vi "Dashboard Main.vi"() -> ()   [LabVIEW 2017]
uses:
  Shared/AutonomousRoutine.ctl
  Shared/RobotPosition.ctl
  Shared/AutoRoutineSelector.ctl
  <vilib>/Rock Robotics/WPI/DriverStation/WPI_DriverStationAllianceInfo.ctl
  <vilib>/Utility/miscctls.llb/LVRowAndColumnTypeDef.ctl
  <vilib>/event_ctls.llb/eventvkey.ctl
  <vilib>/Rock Robotics/Network Tables/NT Read Numeric Array.vi
  <vilib>/Rock Robotics/WPI/Dashboard/WPI_DashboardLogging Global.vi
  <vilib>/Rock Robotics/Network Tables/NT Write Boolean.vi
  <vilib>/Rock Robotics/Network Tables/NT Write Numeric Array.vi
panel:
  in  "Camera Settings Right":T1={"Frame Rate"=30, "Compression"=30, "Size"=1, "DB Camera Config"=FALSE} {"Frame Rate" scale=1.0..30.0; "Compression" scale=100.0..-1.0; "Size" items=["640x480", "320x240", "160x120"]}
  in  "Camera Name Right":string(combo)="No Camera Selection"
  out "Camera Info":cluster{"Mbps LED":bool, "Mbps":dbl, "fps":dbl} {"fps" format="%#.1g"; "Mbps" format="%#.1g"}
  in  "Camera Settings":T1={"Frame Rate"=30, "Compression"=30, "Size"=1, "DB Camera Config"=FALSE} {"Frame Rate" scale=1.0..30.0; "Compression" scale=100.0..-1.0; "Size" items=["640x480", "320x240", "160x120"]}
  in  "TCP":refnum<k5>
  in  "Rec Mode":enum32{"Stop", "Record", "Playback"}(radio)
  out "Robot IP":string
  out "Image Message":string="Timeout in Camera Communications"
  in  "Dashboard Tab":T2(tab)
  in  "Select Auto":string(combo)="Select Autonomous ..."
  out "NT Connection":bool
  out "MotorChart R":cluster{"Numeric":dbl, "Numeric":dbl}(graph)
  out "MotorChart L":cluster{"Numeric":dbl, "Numeric":dbl}(graph)
  out "MotorSliders R":cluster{"MotorSlide1":dbl, "MotorSlide2":dbl} {"MotorSlide2" scale=-1.0..1.0 scale format="%#_2e"; "MotorSlide1" scale=-1.0..1.0 scale format="%#_2e"}
  out "MotorSliders L":cluster{"MotorSlide1":dbl, "MotorSlide2":dbl} {"MotorSlide2" scale=-1.0..1.0 scale format="%#_2e"; "MotorSlide1" scale=-1.0..1.0 scale format="%#_2e"}
  out "Gyro":dbl(knob) scale=0.0..360.0
  out "JS1 Z":dbl(slide) scale=-1.0..1.0 scale format="%#_2e"
  out "JS1 Graph":cluster{"X":dbl, "Y":dbl}[](graph)
  out "JS1 Buttons":T3
  out "JS2 Z":dbl(slide) scale=-1.0..1.0 scale format="%#_2e"
  out "JS2 Graph":cluster{"X":dbl, "Y":dbl}[](graph)
  out "JS2 Buttons":T3
  out "Mode":T4(ring)=enum."Auto Disabled"
  in  "Battery Number":string
  out "Camera Image Right":T5(plugin-control)
  in  "DB/String 9":string
  in  "DB/String 8":string
  in  "DB/String 7":string
  in  "DB/String 6":string
  in  "DB/String 5":string
  in  "DB/String 4":string
  in  "DB/String 3":string
  in  "DB/String 2":string
  in  "DB/String 1":string
  in  "DB/String 0":string
  in  "DB/Slider 0":dbl(slide) scale=0.0..5.0
  in  "DB/Slider 1":dbl(slide) scale=0.0..5.0
  in  "DB/Slider 2":dbl(slide) scale=0.0..5.0
  in  "DB/Slider 3":dbl(slide) scale=0.0..5.0
  out "DB/LED 3":bool
  out "DB/LED 2":bool
  out "DB/LED 1":bool
  out "DB/LED 0":bool
  in  "DB/Button 3":bool
  in  "DB/Button 2":bool
  in  "DB/Button 1":bool
  in  "DB/Button 0":bool caption="New Name"
  in  "Routine":T6 items=["Definately Switch", "Definately Scale", "Switch if in front, else scale", "Scale if in front, else switch", "Switch if in front, else nothing", "Scale if in front, else nothing", "Drive across line"]
  in  "RR":T7
  in  "RL":T7
  in  "LR":T7
  in  "Position":T8
  in  "LL":T7
  out "Our Right Team Switch":bool
  out "Our Left Team Switch":bool
  out "Center Right Scale":bool
  out "Center Left Scale":bool
  out "Opponent Right Switch":bool
  out "Opponent Left Switch":bool
  in  "Test Slider":dbl(slide) scale=0.0..100.0 scale format="%#_3g"
  in  "On/Off":bool caption="Solenoid"
  in  "Test Name":u16(ring) items=["Select the test to run..."]
  in  "Test Tree":string(tree)
  in  "Motor":cluster{"Value":dbl, "Enable":bool} {"Value" scale=-1.0..1.0 scale format="%#_3g"}
  out "Progress":T9 {"Test Progress" scale=0.0..100.0}
  in  "Rev/Fwd":cluster{"Forward":bool, "Reverse":bool}
  in  "Test Ring":u16(ring) items=["Monochrome", "Color"]
  out "Cmd Status":string
  in  "Execute Command":bool
  in  "Command Params":string[][](table)
  in  "Command Selection":i32(listbox)
  in  "CheckList":i32(listbox)
  out "Tree":string(tree)
  out "Camera Image":T5(plugin-control)
  out "Background":bool
  in  "Camera Name":string(combo)="No Camera Selection"
  # "HW"
  # "HW"
  # "Joysticks"
  # "Drive Motors"
  # "Front"
  # "Right"
  # "Left"
  # "Back"
  # "Opponent Switch"
  # "Center Scale"
  # "Our Team Switch"
  # "1"
  # "2"
  # "3"
  # "4"
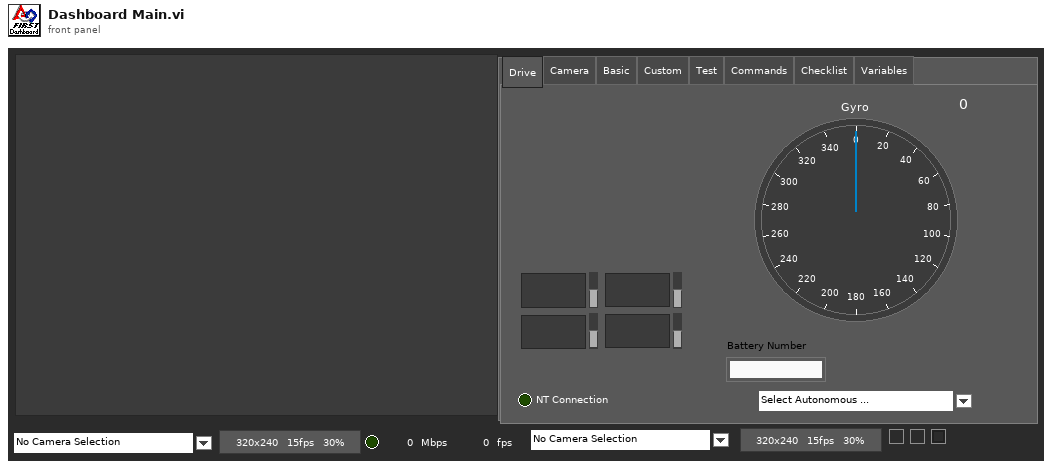
[diagram p1: front panel]
types:
  T1 = cluster{"Frame Rate":i32, "Compression":i32, "Size":u16, "DB Camera Config":bool}
  T2 = enum32{"Drive", "Camera", "Basic", "Custom", "Test", "Commands", "Checklist", "Variables"}
  T3 = cluster{bool, bool, bool, bool, bool, bool, bool, bool, bool, bool, bool, bool}
  T4 = enum8{"Tele-Op Disabled", "Tele-Op Enabled", "Auto Disabled", "Auto Enabled", "Test Disabled", "Test Enabled", "Disconnected", "No Code", "E-Stop"}
  T5 = typedef "IMAQ Image.ctl" = refnum<image>
  T6 = typedef "AutoRoutineSelector.ctl" = u16
  T7 = typedef "AutonomousRoutine.ctl" = enum16{"Score Scale", "Score Switch"}
  T8 = typedef "RobotPosition.ctl" = enum16{"1", "2", "3", "4"}
  T9 = cluster{"Test Progress":u8, "Test Progress Text":string}
  T10 = cluster{"Save Path":path, "Interval (s)":dbl, "Keep":i32}
  T11 = typedef "Image Type" = u32
  T12 = cluster{"IDs":cluster{"RPC field ID":u16, "Unique ID":u16}, "String":string}
  T13 = cluster{"Error Strings":string, "Disable Counts":cluster{u16, u16}, "Rail Faults":cluster{u16, u16, u16}, "Robot IP":string, "DB Mode":u8, "Event Info":cluster{"Name":string, "Type":u8, "Number":u16, "Replay":u8}}
  T14 = cluster{"Storage":cluster{"Disk Free":u64, "RAM Block":u32, "RAM free":u32}, "CPU Utilization":cluster{"CPU % ISR":sgl, "CPU % Time Crit":sgl, "CPU % Timed Str":sgl, "CPU % High":sgl, "CPU % Above":sgl, "CPU % Normal":sgl, "CPU % Low":sgl}, "CAN":cluster{"% Bus Utilization":sgl, "Bus Off Cnt":u32, "TX_FIFO Full Cnt":u32, "Receive Error Cnt":u8, "Transmit Error Cnt":u8}, "HID":cluster{"HID Outputs":u32, "Rumble Low":u16, "Rumble High":u16}[]}
  T15 = cluster{"Status bits":cluster{"Test Mode":bool, "Autonomous":bool, "Enabled":bool, "Code Start":bool, "Brownout":bool, "Reserved 2":bool, "Reserved 3":bool, "E-Stop":bool}, "Code Trace":cluster{"Disabled":bool, "TeleOp":bool, "Auto":bool, "Test":bool}, "Controller Type":enum16{"unknown", "cRIO", "roboRio"}, "Code?":enum16{"unknown", "noCode", "code"}, "Battery V":dbl}
  T16 = cluster{"Control Bits":cluster{"TestMode":bool, "Autonomous":bool, "Enabled":bool, "FMS Present":bool, bool, bool, bool, "E-Stop":bool}, "Team Station ":u8, "Countdown":sgl, "Joystick Values":cluster{"Axes":dbl[], "Buttons":bool[], "POVs":i16[]}[]}
  T17 = cluster{"Axes":dbl[], "Buttons":bool[], "POVs":i16[]}[]
  T18 = cluster{"Axes":dbl[], "Buttons":bool[], "POVs":i16[]}
  T19 = cluster{"Buttons[0]":bool, "Buttons[1]":bool, "Buttons[2]":bool, "Buttons[3]":bool, "Buttons[4]":bool, "Buttons[5]":bool, "Buttons[6]":bool, "Buttons[7]":bool, "Buttons[8]":bool, "Buttons[9]":bool, "Buttons[10]":bool, "Buttons[11]":bool}
  T20 = cluster{"Camera Image":refnum<vi>, "Dashboard Tab":refnum<vi>, "Background":refnum<vi>, "Rec Mode":refnum<vi>, "Test Slider":refnum<vi>, "On/Off ":refnum<vi>, "Test Ring":refnum<vi>, "Rev/Fwd":refnum<vi>, "Test Name":refnum<vi>, "Motor":refnum<vi>, "Progress":refnum<vi>, "CheckList":refnum<vi>, "Tree":refnum<vi>, "Test Tree":refnum<vi>, "Command Params":refnum<vi>, "Command Selection":refnum<vi>, "Execute Command":refnum<vi>, "Cmd Status":refnum<vi>, "Camera Settings":refnum<vi>, "Camera Name":refnum<vi>, "Camera Info":refnum<vi>, "Camera Settings Right":refnum<vi>, "Camera Name Right":refnum<vi>, "Camera Image Right":refnum<vi>}
  T21 = cluster{"Camera Name":string, string, "Saved DB Images Info":cluster{"Save Path":path, "Interval (s)":dbl, "Keep":i32}}
  T22 = cluster{"Camera Name Right":string, string, "Saved DB Images Info":cluster{"Save Path":path, "Interval (s)":dbl, "Keep":i32}}
  T23 = typedef "WPI_DriverStationAllianceInfo.ctl" = enum16{"Red", "Blue", "Invalid"}
  T24 = cluster{"Operation":enum16{"Update", "Clear"}, "Color Box":u32}[]
  T25 = typedef "eventvkey.ctl" = enum16{"ASCII", "Enter", "Return", "Shift", "Ctrl", "Alt", "Cmd", "Opt", "Caps", "NumLock", "Clear", "Break", "Up", "Down", "Left", "Right", "Insert", "Delete", "Home", "End", "PageUp", "PageDown", "Escape", "Help", "Pause", "ScrollLock", "F1", "F2", "F3", "F4", "F5", "F6", "F7", "F8", "F9", "F10", "F11", "F12", "F13", "F14", "F15", "F16", "F17", "F18", "F19", "F20", "F21", "F22", "F23", "F24", "Play", "VolumeUp", "VolumeDown", "Mute", "Two Byte Char"}
  T26 = cluster{"Image Size":bool, "Image Type":bool, "Pixel Value":bool, "ROI Information":bool, "Zoom Factor":bool}
  T27 = cluster{"Operation":enum16{"Update", "Clear"}, "Color Box":u32}
  T28 = typedef "LVRowAndColumnTypeDef.ctl" = cluster{"Row":i32, "Column":i32}
  T29 = cluster{"Shift":bool, "Ctrl":bool, "Alt":bool, "Cmd":bool, "Opt":bool}
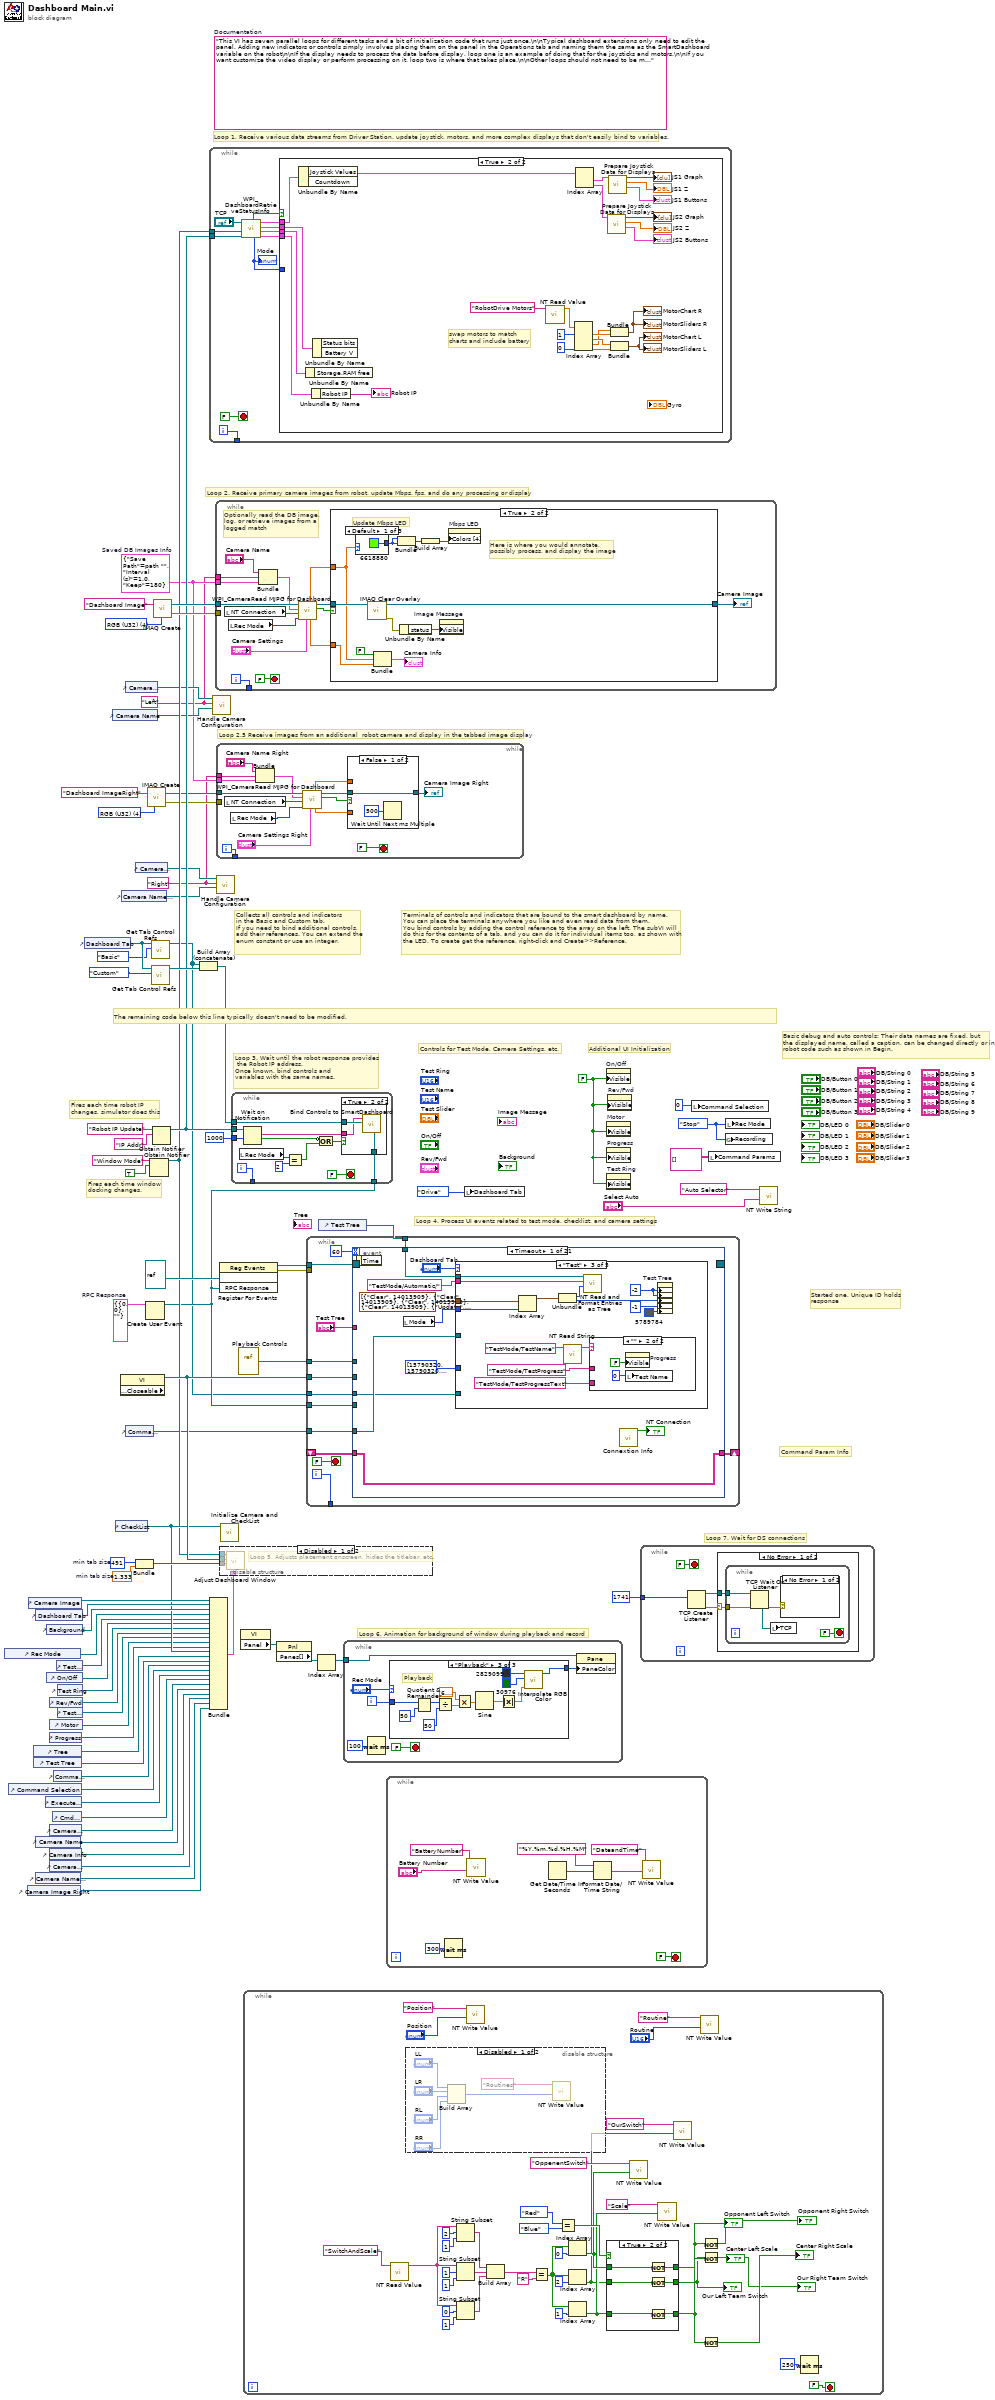
[diagram p0: block diagram]
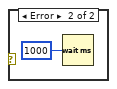
[diagram p6: hidden frame]
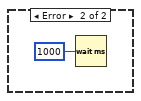
[diagram p7: hidden frame]
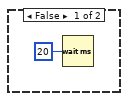
[diagram p8: hidden frame]
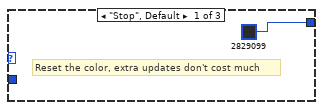
[diagram p9: hidden frame]
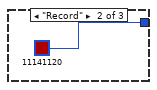
[diagram p10: hidden frame]
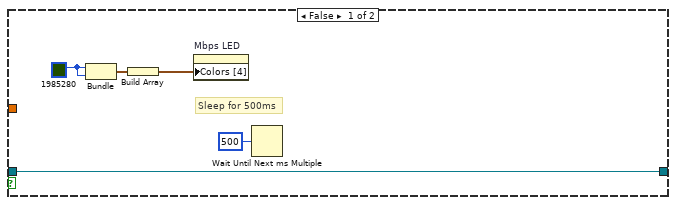
[diagram p12: hidden frame]
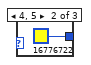
[diagram p13: hidden frame]
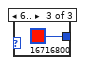
[diagram p14: hidden frame]
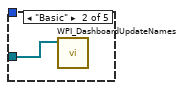
[diagram p16: hidden frame]
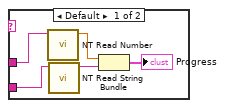
[diagram p17: hidden frame]
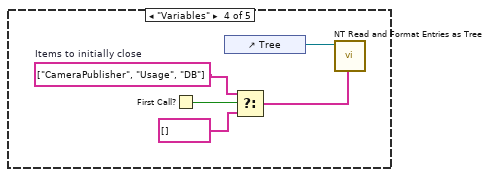
[diagram p18: hidden frame]
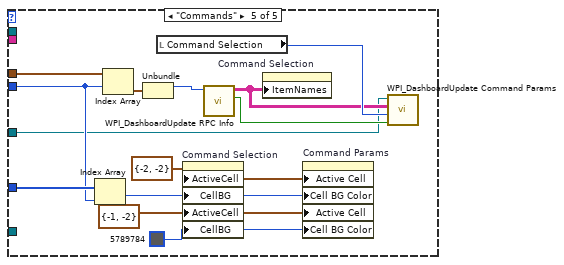
[diagram p19: hidden frame]
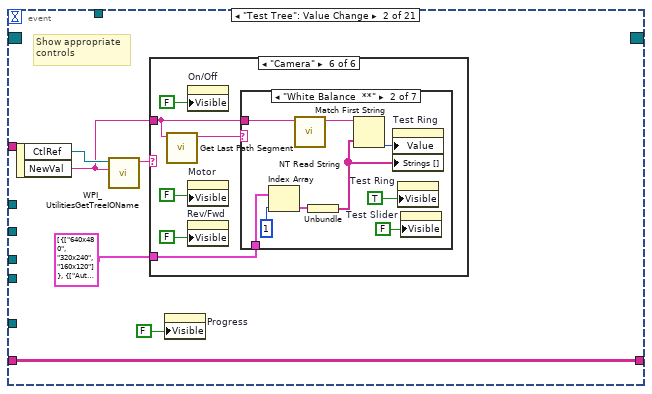
[diagram p20: hidden frame]
diagram:
  w3 = T10 {"Save Path"=path "", "Interval (s)"=1.0, "Keep"=180}  # Saved DB Images Info
  w2 = "Right"
  w1 = "Left"
  w13 = T11 4 items=["Grayscale (U8)", "Grayscale (I16)", "Grayscale (SGL)", "Complex (CSG)", "RGB (U32)", "HSL (U32)", "RGB (U64)"] ("Image Type")
  w29 = T12 {"IDs"={"RPC field ID"=0, "Unique ID"=0}, "String"=""}  # RPC Response
  w52 = 491  # min tab size
  w51 = 1.333  # min tab size
  w59 = enum32{"Stop", "Record", "Playback"}."Stop" ("Rec Mode")
  w36 = FALSE ("Visible")
  (unwired) "This VI has seven parallel loops for different tasks and a bit of initialization code that runs just once.\n\nTypical dashboard extensions only need to edit the panel. Adding new indicators or controls simply involves placing them on the panel in the Operations tab and naming them the same as the SmartDashboard variable on the robot\n\nIf the display needs to process the data before display, loop one is an example of doing that for the joysticks and motors.\n\nIf you want customize the video display or perform processing on it, loop two is where that takes place.\n\nOther loops should not need to be modified. They are pretty standard, and document the task they perform."  # Documentation
  w76 = T11 4 items=["Grayscale (U8)", "Grayscale (I16)", "Grayscale (SGL)", "Complex (CSG)", "RGB (U32)", "HSL (U32)", "RGB (U64)"] ("Image Type")
  # "Loop 2.5 Receive images from an additional  robot camera and display in the tabbed image display"
  # "Command Param Info"
  # "Started one, Unique ID holds\nresponse"
  # "Loop 7. Wait for DS connections"
  # "Basic debug and auto controls: Their data names are fixed, but\nthe displayed name, called a caption, can be changed directly or in\nrobot code such as shown in Begin."
  # "Controls for Test Mode, Camera Settings, etc."
  # "Additional UI Initialization"
  # "Loop 6. Animation for background of window during playback and record"
  # "Fires each time robot IP\nchanges, simulator does this"
  # "Fires each time window\ndocking changes."
  # "Collects all controls and indicators\nin the Basic and Custom tab.\nIf you need to bind additional controls,\nadd their references. You can extend the\nenum constant or use an integer."
  # "The remaining code below this line typically doesn't need to be modified."
  # "Loop 4. Process UI events related to test mode, checklist, and camera settings"
  # "Terminals of controls and indicators that are bound to the smart dashboard by name.\nYou can place the terminals anywhere you like and even read data from them.\nYou bind controls by adding the control reference to the array on the left. The subVI will\ndo this for the contents of a tab, and you can do it for individual items too, as shown with\nthe LED. To create get the reference, right-click and Create>>Reference."
  # "Loop 3. Wait until the robot response provides\n the Robot IP address.\nOnce known, bind controls and\nvariables with the same names."
  # "Loop 1. Receive various data streams from Driver Station, update joystick, motors, and more complex displays that don't easily bind to variables."
  # "Loop 2. Receive primary camera images from robot, update Mbps, fps, and do any processing or display"
  n1 = control-ref of="Rec Mode"() -> (w42:refnum<vi>)
  n2 = control-ref of="Command Selection"() -> (w28:refnum<vi>)
  n3 = control-ref of="Camera Image Right"() -> (w6:refnum<vi>)
  n4 = control-ref of="Camera Image"() -> (w54:refnum<vi>)
  n5 = control-ref of="Tree"() -> (w46:refnum<vi>)
  n6 = control-ref of="Test Tree"() -> (w45:refnum<vi>)
  n7 = control-ref of="Dashboard Tab"() -> (w53:refnum<vi>)
  n8 = control-ref of="Camera Name"() -> (w19:refnum<vi>)
  n9 = control-ref of="Camera Name Right"() -> (w7:refnum<vi>)
  n10 = control-ref of="Execute Command"() -> (w30:refnum<vi>)
  n11 = control-ref of="Background"() -> (w49:refnum<vi>)
  n12 = control-ref of="On/Off"() -> (w40:refnum<vi>)
  n13 = control-ref of="Progress"() -> (w37:refnum<vi>)
  n14 = control-ref of="Camera Settings"() -> (w20:refnum<vi>)
  n15 = control-ref of="Camera Info"() -> (w18:refnum<vi>)
  n16 = control-ref of="Camera Settings Right"() -> (w8:refnum<vi>)
  n17 = control-ref of="Rev/Fwd"() -> (w38:refnum<vi>)
  n18 = control-ref of="Motor"() -> (w43:refnum<vi>)
  n19 = control-ref of="Cmd Status"() -> (w24:refnum<vi>)
  n20 = control-ref of="Command Params"() -> (w31:refnum<vi>)
  n21 = control-ref of="Test Slider"() -> (w41:refnum<vi>)
  n22 = control-ref of="Test Ring"() -> (w39:refnum<vi>)
  n23 = control-ref of="Test Name"() -> (w44:refnum<vi>)
  n24 = control-ref of="Dashboard Tab"() -> (w57:refnum<vi>)
  n25 = control-ref of="Camera Name"() -> (w21:refnum<vi>)
  n26 = control-ref of="CheckList"() -> (w47:refnum<vi>)
  n27 = property class="VI" props=["Front Panel.Closeable"]() -> (reference out=w58:refnum<vi>)  [unwired: 2 in, 2 out]
  n28 = control-ref of="Camera Name Right"() -> (w9:refnum<vi>)
  n29 = control-ref of="Camera Settings"() -> (w22:refnum<vi>)
  n30 = control-ref of="Command Params"() -> (w23:refnum<vi>)
  n31 = control-ref of="Camera Settings Right"() -> (w10:refnum<vi>)
  n32 = Bundle("min tab size"=w52, "min tab size"=w51) -> (w50:cluster{"min tab size":i32, "min tab size":dbl})  [unwired: 1 in]
  n33 = Create User Event(user event datatype=w29) -> (user event=w25:refnum<user-event>)  [unwired: 1 in, 1 out]
  n34 = call "IMAQ Create"("Image Name"="Dashboard ImageRight", "Image Type"=w13) -> ("New Image"=w12:T5, "error out"=w11:errorcluster)  [unwired: 2 in, 1 out]
  n35 = Obtain Notifier(name (unnamed)="Window Mode", notification data type=TRUE) -> (notifier out=w34:refnum<notifier>)  [unwired: 2 in, 2 out]
  n36 = call <vilib>:"Get Tab Control Refs.vi"("Page Index"=T2."Basic" ("Dashboard Tab"), "TabControl in"=w57) -> ("ControlsOnPage"=w17:refnum<vi>[])  [unwired: 9 in]
  n37 = call <vilib>:"Get Tab Control Refs.vi"("Page Index"=T2."Custom" ("Dashboard Tab"), "TabControl in"=w57) -> ("ControlsOnPage"=w56:refnum<vi>[])  [unwired: 9 in]
  n38 = Obtain Notifier(name (unnamed)="Robot IP Update", notification data type="IP Addr" ("name (unnamed)")) -> (notifier out=w35:refnum<notifier>)  [unwired: 2 in, 2 out]
  n39 = call "IMAQ Create"("Image Name"="Dashboard Image", "Image Type"=w76) -> ("New Image"=w74:T5, "error out"=w73:errorcluster)  [unwired: 2 in, 1 out]
  n40 = Build Array (concatenate)(w17, w56) -> (w55:refnum<vi>[])
  n41 = while {
    tunnel: [w86] -> _
    tunnel: w35 -> [w80]
    tunnel: w34 -> [w77]
    i -> [w86]
    stop <- FALSE stop-if-true
    n42 = call <vilib>:"WPI_DashboardRetrieveStatusInfo.vi"("Binding Refnum"=w80, "Window Mode Notifier"=w77, "TCP Cnx"="TCP") -> ("Power and Errors"=w81:T13, "Robot Metrics"=w84:T14, "Status Info"=w85:T15, "Control Info"=w82:T16, "Robot Mode"=w79:T4, "Process?"=w83:bool)  [unwired: 3 in]
    "Mode" <- w79
    n43 = case shown="True" w83 {
      tunnel: w85 -> [_ w112]
      tunnel: w84 -> [_ w111]
      tunnel: w82 -> [_ w110]
      tunnel: w81 -> [_ w109]
      tunnel: w79 -> [_ _]
      frame False {
        n44 = Wait (ms)(milliseconds to wait=u32 20) -> ()  [unwired: 1 out]
      }
      frame True {
        # "swap motors to match\ncharts and include battery"
        n45 = Unbundle By Name(w110) -> ("Joystick Values"=w100:T17)  [unwired: 1 out]
        n46 = Unbundle By Name(w111) -> ()  [unwired: 1 out]
        n47 = Unbundle By Name(w109) -> ("Robot IP"=→"Robot IP":string)
        n48 = Unbundle By Name(w112) -> ()  [unwired: 2 out]
        n49 = call-poly <vilib>:"NT Read Value.vi"("Name"="RobotDrive Motors") -> ("Numeric Array"=w90:dbl[])  [unwired: 9 in, 1 out]
        n50 = Index Array(array=w90, index #1=1, index #4=0) -> (element #1=w104:dbl, element #2=w105:dbl, element #3=w103:dbl, element #4=w108:dbl)  [unwired: 2 in]
        n51 = Index Array(array=w100) -> (element #1=w99:T18, element #2=w95:T18)  [unwired: 2 in]
        n52 = call "Prepare Joystick Data for Displays.vi"("Joystick Values"=w95) -> ("Buttons"=→"JS2 Buttons":T19, "Z Axis"=→"JS2 Z":dbl, "Cartesian Data"=→"JS2 Graph":cluster{"X axis":dbl, "X axis":dbl}[])  [unwired: 8 in]
        n53 = call "Prepare Joystick Data for Displays.vi"("Joystick Values"=w99) -> ("Buttons"=→"JS1 Buttons":T19, "Z Axis"=→"JS1 Z":dbl, "Cartesian Data"=→"JS1 Graph":cluster{"X axis":dbl, "X axis":dbl}[])  [unwired: 8 in]
        n54 = Bundle("Numeric"=w103, "Numeric"=w104) -> (→"MotorChart R" →"MotorSliders R":cluster{"Numeric":dbl, "Numeric":dbl})  [unwired: 1 in]
        n55 = Bundle("Numeric"=w105, "Numeric"=w108) -> (→"MotorChart L" →"MotorSliders L":cluster{"Numeric":dbl, "Numeric":dbl})  [unwired: 1 in]
      }
    }
  }
  n56 = Bundle("Camera Image"=w54, "Dashboard Tab"=w53, "Background"=w49, "Rec Mode"=w42, "Test Slider"=w41, "On/Off"=w40, "Test Ring"=w39, "Rev/Fwd"=w38, "Test Name"=w44, "Motor"=w43, "Progress"=w37, "CheckList"=w47, "Tree"=w46, "Test Tree"=w45, "Command Params"=w31, "Command Selection"=w28, "Execute Command"=w30, "Cmd Status"=w24, "Camera Settings"=w20, "Camera Name"=w19, "Camera Info"=w18, "Camera Settings Right"=w8, "Camera Name Right"=w7, "Camera Image Right"=w6) -> (w48:T20)  [unwired: 1 in]
  n57 = call "Handle Camera Configuration.vi"("CameraNameRef"=w21, "Display Name"=w1, "ClusterRef"=w22) -> ()  [unwired: 9 in]
  n58 = while {
    tunnel: w74 -> [w125]
    tunnel: w73 -> [_]
    tunnel: [w126] -> _
    tunnel: w3 -> [w116]
    tunnel: w1 -> [w113]
    i -> [w126]
    stop <- FALSE stop-if-true
    # "Optionally read the DB image,\nlog, or retrieve images from a\nlogged match"
    n59 = local read "NT Connection"() -> (w117:bool)
    n60 = local read "Rec Mode"() -> (w121:enum32{"Stop", "Record", "Playback"})
    n61 = Bundle("Camera Name"="Camera Name", w113, "Saved DB Images Info"=w116) -> (w115:T21)  [unwired: 1 in]
    n62 = call <vilib>:"WPI_CameraRead MJPG for Dashboard.vi"("Camera Settings"="Camera Settings", "Rec Mode"=w121, "NT Connection"=w117, "Capture Info"=w115, "Refnum in"=w125) -> ("Active"=w123:bool, "Refnum out"=w124:T5, "FPS"=w122:dbl, "Bandwidth (Mbps)"=w120:dbl)  [unwired: 3 in]
    n63 = case shown="True" w123 {
      tunnel: w124 -> [w128 w139]
      tunnel: w120 -> [_ w136]
      tunnel: w122 -> [_ w137]
      tunnel: [w128 w133] -> w118
      frame False {
        w130 = u32 1985280 ("Color Box")
        # "Sleep for 500ms"
        n64 = Bundle("Color Box"=w130, "Color Box"=w130) -> (w131:cluster{"Color Box":u32, "Color Box":u32})  [unwired: 1 out]
        n65 = Build Array(w131) -> (w129:cluster{"Color Box":u32, "Color Box":u32}[])
        n66 = property on="Mbps LED" class="Bool (strict)"("Colors [4]"=w129) -> ()  [unwired: 2 in, 2 out]
        n67 = Wait Until Next ms Multiple(millisecond multiple=u32 500) -> ()  [unwired: 1 out]
      }
      frame True {
        # "Here is where you would annotate,\npossibly process, and display the image"
        # "Update Mbps LED"
        n68 = case shown="Default" w136 {
          tunnel: [u32 6618880 ("Color Box") u32 16776722 ("Color Box") u32 16716800 ("Color Box")] -> w140
          frame Default {
          }
          frame 4, 5 {
          }
          frame 6.. {
          }
        }
        n69 = call "IMAQ Clear Overlay"("Image"=w139) -> ("error out"=w142:errorcluster, "Image Out"=w133:T5)  [unwired: 2 in, 7 out]
        n70 = Bundle(FALSE, "Bandwidth (Mbps)"=w136, "FPS"=w137) -> (→"Camera Info":cluster{bool, "Bandwidth (Mbps)":dbl, "FPS":dbl})  [unwired: 1 in]
        n71 = Bundle("Color Box"=w140, "Color Box"=w140) -> (w141:cluster{"Color Box":u32, "Color Box":u32})  [unwired: 1 out]
        n72 = Unbundle By Name(w142) -> ("status"=w143:bool)
        n73 = Build Array(w141) -> (w138:cluster{"Color Box":u32, "Color Box":u32}[])
        n74 = property on="Image Message" class="Str"("Visible"=w143) -> ()  [unwired: 2 in, 2 out]
        n75 = property on="Mbps LED" class="Bool (strict)"("Colors [4]"=w138) -> ()  [unwired: 2 in, 2 out]
      }
    }
    "Camera Image" <- w118
  }
  n76 = call "Handle Camera Configuration.vi"("CameraNameRef"=w9, "Display Name"=w2, "ClusterRef"=w10) -> ()  [unwired: 9 in]
  n77 = while {
    tunnel: w12 -> [w161]
    tunnel: w11 -> [_]
    tunnel: [w156] -> _
    tunnel: w3 -> [w150]
    tunnel: w2 -> [w147]
    i -> [w156]
    stop <- FALSE stop-if-true
    n78 = local read "NT Connection"() -> (w151:bool)
    n79 = local read "Rec Mode"() -> (w160:enum32{"Stop", "Record", "Playback"})
    n80 = Bundle("Camera Name Right"="Camera Name Right", w147, "Saved DB Images Info"=w150) -> (w149:T22)  [unwired: 1 in]
    n81 = call <vilib>:"WPI_CameraRead MJPG for Dashboard.vi"("Camera Settings"="Camera Settings Right", "Rec Mode"=w160, "NT Connection"=w151, "Capture Info"=w149, "Refnum in"=w161) -> ("Active"=w155:bool, "Refnum out"=w158:T5, "FPS"=w153:dbl, "Bandwidth (Mbps)"=w154:dbl)  [unwired: 3 in]
    n82 = case shown="False" w155 {
      tunnel: w158 -> [w162 w164]
      tunnel: w154 -> [_ _]
      tunnel: w153 -> [_ _]
      tunnel: [w162 w164] -> w152
      frame False {
        n83 = Wait Until Next ms Multiple(millisecond multiple=u32 500) -> ()  [unwired: 1 out]
      }
      frame True {
      }
    }
    "Camera Image Right" <- w152
  }
  n84 = register-events(refnum<vi> refnum, w25) -> (reference out=w63:refnum<event-registration>, error out=w62:errorcluster)  [unwired: 2 in]
  n85 = disable-structure shown="Disabled" {
    disable-tunnel: w58 -> [w168 _]
    disable-tunnel: w50 -> [w167 _]
    disable-tunnel: w48 -> [w166 _]
    disable-tunnel: w34 -> [w165 _]
    frame Disabled {
      # "Loop 5. Adjusts placement onscreen, hides the titlebar, etc."
      n86 = call "Adjust Dashboard Window.vi"("Sizing Refnums"=w166, "Size Constraints"=w167, "VI"=w168, "WIn Mode"=w165) -> ()  [unwired: 8 in]
    }
    frame Enabled {
    }
  }
  n87 = call "Initialize Camera and CheckList.vi"("ListBox in"=w47) -> ()  [unwired: 11 in]
  n88 = while {
    tunnel: w55 -> [w180]
    tunnel: w35 -> [w178]
    tunnel: [w176] -> _
    tunnel: u32 1000 ("milliseconds to wait") -> [w175]
    tunnel: w25 -> [w169]
    i -> [w176]
    stop <- FALSE stop-if-true
    n89 = local read "Rec Mode"() -> (w171:enum32{"Stop", "Record", "Playback"})
    n90 = Wait on Notification(notifier=w178, timeout in ms (-1)=w175) -> (notification=w177:string, timed out?=w173:bool)  [unwired: 2 in, 2 out]
    n91 = Equal?(x=w171, y=u16 2 ("Rec Mode")) -> (x = y?=w172:bool)
    n92 = Compound Arithmetic op=OR(invert w173, w172) -> (w174:bool)
    n93 = case shown="True" w174 {
      tunnel: w180 -> [_ w183]
      tunnel: w177 -> [_ w182]
      tunnel: w169 -> [_ w181]
      frame False {
      }
      frame True {
        n94 = call <vilib>:"Bind Controls to SmartDashboard.vi"("RPC ref"=w181, "Bound Control Refs"=w183, "Server IP Address"=w182) -> ()  [unwired: 9 in]
      }
    }
  }
  n95 = vi-ref "Playback Controls.vi"() -> (w64:refnum<vi>)
  n96 = property class="VI"() -> ("Panel"=w66:refnum<vi>)  [unwired: 2 in, 2 out]
  n97 = while {
    stop <- FALSE stop-if-true
    n98 = call-poly <vilib>:"NT Read Value.vi"("Name"="SwitchAndScale") -> ("String"=w184:string)  [unwired: 9 in, 1 out]
    n99 = disable-structure shown="Disabled" {
      frame Disabled {
        n100 = Build Array("LL", "LR", "RL", "RR") -> (w225:T7[])
        n101 = call-poly <vilib>:"NT Write Value.vi"("Numeric Array"=w225, "Name"="Routines") -> ()  [unwired: 9 in, 1 out]
      }
      frame Enabled {
      }
    }
    n102 = String Subset(string=w184, offset (0)=2, length (rest)=1 ("length (rest)")) -> (substring=w214:string)
    n103 = String Subset(string=w184, offset (0)=1, length (rest)=1 ("length (rest)")) -> (substring=w213:string)
    n104 = String Subset(string=w184, offset (0)=0, length (rest)=1 ("length (rest)")) -> (substring=w212:string)
    n105 = call-poly <vilib>:"NT Write Value.vi"("Numeric"="Position", "Name"="Position") -> ()  [unwired: 9 in, 1 out]
    n106 = Build Array(w214, w213, w212) -> (w211:string[])
    n107 = Equal?(x=w211, y="R") -> (x = y?=w206:bool[])
    n108 = Equal?(x=WPI_DriverStationAllianceInfo."Red" ("y"), y=WPI_DriverStationAllianceInfo."Blue") -> (x = y?=w202:bool)
    n109 = Index Array(array=w206, index=0) -> (element=w192:bool)
    n110 = Index Array(array=w206, index=2) -> (element=w190:bool)
    n111 = Index Array(array=w206, index=1) -> (element=w191:bool)
    n112 = case shown="True" w202 {
      tunnel: w190 -> [w228 w232]
      tunnel: [w228 w231] -> w197
      tunnel: w191 -> [w230 w234]
      tunnel: [w230 w233] -> w200
      tunnel: w192 -> [w229 w236]
      tunnel: [w229 w235] -> w198
      frame False {
      }
      frame True {
        n113 = Not(x=w236) -> (.not. x?=w235:bool)
        n114 = Not(x=w232) -> (.not. x?=w231:bool)
        n115 = Not(x=w234) -> (.not. x?=w233:bool)
      }
    }
    "Opponent Left Switch" <- w198
    "Center Left Scale" <- w200
    "Our Left Team Switch" <- w197
    n116 = call-poly <vilib>:"NT Write Value.vi"("Boolean"=w192, "Name"="OppenentSwitch") -> ()  [unwired: 9 in, 1 out]
    n117 = call-poly <vilib>:"NT Write Value.vi"("Boolean"=w191, "Name"="Scale") -> ()  [unwired: 9 in, 1 out]
    n118 = call-poly <vilib>:"NT Write Value.vi"("Boolean"=w190, "Name"="OurSwitch") -> ()  [unwired: 9 in, 1 out]
    n119 = call-poly <vilib>:"NT Write Value.vi"("Numeric"="Routine", "Name"="Routine") -> ()  [unwired: 9 in, 1 out]
    n120 = Not(x=w198) -> (.not. x?=→"Opponent Right Switch":bool)
    n121 = Not(x=w197) -> (.not. x?=→"Our Right Team Switch":bool)
    n122 = Not(x=w200) -> (.not. x?=→"Center Right Scale":bool)
    n123 = Wait (ms)(milliseconds to wait=u32 250) -> ()  [unwired: 1 out]
  }
  n124 = property class="Pnl"(reference=w66) -> ("Panes[]"=w67:refnum<vi>[])  [unwired: 1 in, 2 out]
  n125 = Index Array(array=w67) -> (element=w65:refnum<vi>)  [unwired: 1 in]
  n126 = control-ref of="Test Tree"() -> (w68:refnum<vi>)
  n127 = while {
    tunnel: [w246] -> _
    tunnel: w68 -> [w245]
    tunnel: w64 -> [w244]
    tunnel: w63 -> [w243]
    tunnel: w62 -> [_]
    tunnel: w58 -> [w242]
    tunnel: w25 -> [w241]
    tunnel: w23 -> [w240]
    shift-right: [w239] -> _
    shift-left: _ -> [w238]
    tunnel: w17 -> [w237]
    i -> [w246]
    stop <- FALSE stop-if-true
    n128 = event shown="[0] Timeout" {
      selector: w243 -> [_ _ _ _ _ _ _ _ _ _ _ _ _ _ _ _ _ _ _ _ _]
      dyn-events: [_ _ _ _ _ _ _ _ _ _ _ _ _ _ _ _ w506 _ _ _ _] -> _
      timeout: u32 60 ("milliseconds to wait") -> [_ _ _ _ _ _ _ _ _ _ _ _ _ _ _ _ _ _ _ _ _]
      tunnel: w245 -> [w258 _ _ _ _ _ _ _ _ _ _ _ _ _ _ _ _ _ _ _ _]
      tunnel: "Test Tree" -> [_ _ _ _ _ _ _ _ _ _ _ w473 w481 w483 w487 w495 _ _ _ _ _]
      tunnel: w244 -> [_ _ _ _ _ _ _ _ _ _ _ _ _ _ _ _ w508 _ w526 _ _]
      tunnel: w242 -> [_ _ _ _ _ _ _ _ _ _ _ _ _ _ _ _ w504 _ _ _ _]
      tunnel: w241 -> [_ _ _ _ _ _ _ _ _ _ _ _ _ _ _ _ w502 _ _ _ _]
      tunnel: w240 -> [w253 _ _ _ _ _ w424 _ _ _ _ _ _ _ _ _ _ _ _ _ _]
      tunnel: [w252 w301 w403 w408 w417 w421 w422 w431 w441 w448 w460 w472 w479 w482 w486 w494 w501 w521 w523 w527 w540] -> w239
      tunnel: w238 -> [w252 w301 w403 w408 w417 w421 w422 _ _ w448 w460 w472 w479 w482 w486 w494 w501 w521 w523 w527 w540]
      tunnel: w237 -> [w250 _ _ _ _ _ _ _ _ _ _ _ _ _ _ _ _ _ _ _ _]
      event Timeout {
        n129 = event-data() -> ()  [unwired: 1 in, 1 out]
        n130 = local read "Mode"() -> (w255:T4)
        n131 = case shown="\"Test\"" "Dashboard Tab" {
          tunnel: w258 -> [_ _ w274 _ _]
          tunnel: "TestMode/Automatic/" ("Name Pattern") -> [_ _ w273 _ _]
          tunnel: T24 [{"Operation"=enum."Clear", "Color Box"=14013909}, {"Operation"=enum."Clear", "Color Box"=14013909}, {"Operation"=enum."Clear", "Color Box"=14013909}, {"Operation"=enum."Clear", "Color Box"=14013909}, {"Operation"=enum."Update", "Color Box"=14013909}, {"Operation"=enum."Update", "Color Box"=16777215}, {"Operation"=enum."Clear", "Color Box"=14013909}, {"Operation"=enum."Clear", "Color Box"=14013909}, {"Operation"=enum."Clear", "Color Box"=14013909}] -> [_ _ w266 _ w294]
          tunnel: w255 -> [_ _ w265 _ w293]
          tunnel: u32[] [15790320, 15790320, 15790320, 15790320, 16777215, 16777215, 15790320, 15790320, 15790320] -> [_ _ _ _ w299]
          tunnel: w253 -> [_ _ _ _ w287]
          tunnel: w250 -> [_ w260 _ _ _]
          frame "Custom", Default {
          }
          frame "Basic" {
            n132 = call <vilib>:"WPI_DashboardUpdateNames.vi"("Controls on Tab"=w260) -> ()  [unwired: 11 in]
          }
          frame "Test" {
            w272 = -2 ("Active Item:Row Number")
            n133 = Index Array(array=w266, index=w265) -> (element=w267:T27)
            n134 = Unbundle(w267) -> ("Operation"=w268:enum16{"Update", "Clear"}, "Color Box"=w269:u32)
            n135 = call <vilib>:"NT Read String.vi"("Name"="TestMode/TestName") -> ("String"=w263:string)  [unwired: 9 in, 1 out]
            n136 = call <vilib>:"NT Read and Format Entries as Tree.vi"("Operation"=w268, "Name Pattern"=w273, "Tree Refnum"=w274) -> ()  [unwired: 7 in, 2 out]
            n137 = case shown="\"\"" w263 {
              tunnel: "TestMode/TestProgress" ("Name") -> [w276 _]
              tunnel: "TestMode/TestProgressText" ("Name") -> [w275 _]
              frame Default {
                n138 = call <vilib>:"NT Read Number.vi"("Name"=w276) -> ("Numeric"=w277:dbl)  [unwired: 9 in, 1 out]
                n139 = call <vilib>:"NT Read String.vi"("Name"=w275) -> ("String"=w278:string)  [unwired: 9 in, 1 out]
                n140 = Bundle("Numeric"=w277, "String"=w278) -> (→"Progress":cluster{"Numeric":dbl, "String":string})  [unwired: 1 in]
              }
              frame "" {
                n141 = property on="Progress" class="Clust (strict)"("Visible"=FALSE) -> ()  [unwired: 2 in, 2 out]
                n142 = local write "Test Name"(u16 0) -> ()
              }
            }
            n143 = property on="Test Tree" class="Tree (strict)"("Active Item Row Number"=w272, "ActiveColNum"=w272, "CellBG"=w269, "Active Item Row Number"=-1 ("Active Item:Row Number"), "CellBG"=u32 5789784 ("Color Box")) -> ()  [unwired: 2 in, 2 out]
          }
          frame "Variables" {
            w284 = string[] ["CameraPublisher", "Usage", "DB"]  # Items to initially close
            n144 = First Call?() -> (First Call?: T/F=w285:bool)
            n145 = control-ref of="Tree"() -> (w286:refnum<vi>)
            n146 = Select(t=w284, s=w285, f=string[] []) -> (s? t:f=w282:string[])
            n147 = call <vilib>:"NT Read and Format Entries as Tree.vi"("Tags to  Close"=w282, "Tree Refnum"=w286) -> ()  [unwired: 8 in, 2 out]
          }
          frame "Commands" {
            w295 = u32 5789784 ("Color Box")
            w296 = T28 {"Row"=-1, "Column"=-2} ("Active Cell:Active Cell")
            w298 = T28 {"Row"=-2, "Column"=-2} ("Active Cell:Active Cell")
            n148 = Index Array(array=w299, index=w293) -> (element=w297:u32)
            n149 = Index Array(array=w294, index=w293) -> (element=w292:T27)
            n150 = Unbundle(w292) -> ("Operation"=w291:enum16{"Update", "Clear"})  [unwired: 1 out]
            n151 = local read "Command Selection"() -> (w290:i32)
            n152 = property on="Command Selection" class="MCListbox (strict)"("ActiveCell"=w298, "CellBG"=w297, "ActiveCell"=w296, "CellBG"=w295) -> ()  [unwired: 2 in, 2 out]
            n153 = call <vilib>:"WPI_DashboardUpdate RPC Info.vi"("Operation"=w291) -> ("update"=w289:bool, "commands"=w288:string[][])  [unwired: 9 in]
            n154 = property on="Command Selection" class="MCListbox (strict)"("ItemNames"=w288) -> ()  [unwired: 2 in, 2 out]
            n155 = property on="Command Params" class="Tbl (strict)"("Active Cell"=w298, "Cell BG Color"=w297, "Active Cell"=w296, "Cell BG Color"=w295) -> ()  [unwired: 2 in, 2 out]
            n156 = call <vilib>:"WPI_DashboardUpdate Command Params.vi"("Update"=w289, "NewVal"=w290, "Commands"=w288, "Param Tbl"=w287) -> ()  [unwired: 7 in, 1 out]
          }
        }
        n157 = call <vilib>:"Connextion Info.vi"() -> ("Connected"=→"NT Connection":bool)  [unwired: 10 in, 1 out]
      }
      event "Test Tree": Value Change {
        # "Show appropriate\ncontrols"
        n158 = event-data() -> ("CtlRef"=w304:refnum<vi>, "NewVal"=w302:string)  [unwired: 1 in]
        n159 = call <vilib>:"WPI_UtilitiesGetTreeIOName.vi"("NewVal"=w302, "TreeControl in"=w304) -> ("I/O Name"=w305:string)  [unwired: 9 in]
        n160 = case shown="\"Camera\"" w305 {
          selector: w305 -> [_ w312 _ w334 w343 _]
          tunnel: w302 -> [_ _ w331 w333 _ w350]
          tunnel: cluster{string[]}[] [{["640x480", "320x240", "160x120"]}, {["Auto", "Fixed indoor", "Fixed outdoor 1", "Fixed outdoor 2", "Fixed fluorescent 1", "Fixed fluorescent 2", "Hold current"]}, {["Auto", "Flicker-free 50 Hz", "Flicker-free 60 Hz", "Hold current"]}, {["None", "Prioritize frame rate", "Prioritize image quality"]}, {["Monochrome", "Color"]}] -> [_ _ _ _ _ w349]
          frame Default {
            w307 = FALSE ("Visible")
            w306 = FALSE ("Visible")
            n161 = property on="Motor" class="Clust (strict)"("Visible"=w306) -> ()  [unwired: 2 in, 2 out]
            n162 = property on="Test Ring" class="Ring (strict)"("Visible"=w306) -> ()  [unwired: 2 in, 2 out]
            n163 = property on="Rev/Fwd" class="Clust (strict)"("Visible"=w307) -> ()  [unwired: 2 in, 2 out]
            n164 = property on="On/Off" class="Bool (strict)"("Visible"=w307) -> ()  [unwired: 2 in, 2 out]
            n165 = property on="Test Slider" class="Slide (strict)"("Visible"=w307) -> ()  [unwired: 2 in, 2 out]
          }
          frame "Analog Out", "Motor", "PWM" {
            w313 = FALSE ("Visible")
            n166 = case shown="\"Analog Out\"" w312 {
              tunnel: [1.0 ("Value") -1.0 ("Value") 0.0 ("Value")] -> w311
              tunnel: [255.0 ("Value") 1.0 ("Value") 5.0 ("Value")] -> w310
              tunnel: [128.0 ("Value") 0.0 ("Value") 0.0 ("Value")] -> w309
              tunnel: [64.0 ("Value") 0.5 ("Value") 1.0 ("Value")] -> w308
              frame "PWM" {
              }
              frame "Motor", Default {
              }
              frame "Analog Out" {
              }
            }
            n167 = property on="Motor" class="Clust (strict)"("Visible"=TRUE) -> ()  [unwired: 2 in, 2 out]
            n168 = property on="Value" class="Slide (strict)"("Value"=w309, "Scale.Minimum"=w311, "Scale.Maximum"=w310, "Scale.Increment"=w308) -> ()  [unwired: 2 in, 2 out]
            n169 = property on="On/Off" class="Bool (strict)"("Visible"=w313) -> ()  [unwired: 2 in, 2 out]
            n170 = property on="Test Slider" class="Slide (strict)"("Visible"=w313) -> ()  [unwired: 2 in, 2 out]
            n171 = property on="Test Ring" class="Ring (strict)"("Visible"=w313) -> ()  [unwired: 2 in, 2 out]
            n172 = property on="Rev/Fwd" class="Clust (strict)"("Visible"=w313) -> ()  [unwired: 2 in, 2 out]
          }
          frame "Servo" {
            w329 = FALSE ("Visible")
            n173 = call <vilib>:"NT Read Number.vi"("Name"=w331) -> ("Numeric"=w330:dbl)  [unwired: 9 in, 1 out]
            n174 = property on="Test Slider" class="Slide (strict)"("Visible"=TRUE, "Scale.Maximum"=170.0 ("Scale.Range:Maximum")) -> ()  [unwired: 2 in, 2 out]
            n175 = local write "Test Slider"(w330) -> ()
            n176 = property on="Motor" class="Clust (strict)"("Visible"=w329) -> ()  [unwired: 2 in, 2 out]
            n177 = property on="Rev/Fwd" class="Clust (strict)"("Visible"=w329) -> ()  [unwired: 2 in, 2 out]
            n178 = property on="On/Off" class="Bool (strict)"("Visible"=w329) -> ()  [unwired: 2 in, 2 out]
            n179 = property on="Test Ring" class="Ring (strict)"("Visible"=w329) -> ()  [unwired: 2 in, 2 out]
          }
          frame "Relay", "Solenoid" {
            w332 = FALSE ("Visible")
            n180 = property on="Motor" class="Clust (strict)"("Visible"=w332) -> ()  [unwired: 2 in, 2 out]
            n181 = property on="Test Slider" class="Slide (strict)"("Visible"=w332) -> ()  [unwired: 2 in, 2 out]
            n182 = Search and Replace String(input string=w333, search string="/Value  **", replace string="/Direction") -> (result string=w339:string)  [unwired: 5 in, 3 out]
            n183 = property on="Test Ring" class="Ring (strict)"("Visible"=w332) -> ()  [unwired: 2 in, 2 out]
            n184 = call <vilib>:"NT Read String.vi"("Name"=w339) -> ("String"=w337:string)  [unwired: 9 in, 1 out]
            n185 = Equal?(x="Both directions", y=w337) -> (x = y?=w335:bool)
            n186 = Not(x=w335) -> (.not. x?=w336:bool)
            n187 = property on="Rev/Fwd" class="Clust (strict)"("Visible"=w335) -> ()  [unwired: 2 in, 2 out]
            n188 = property on="On/Off" class="Bool (strict)"("Visible"=w336, "Caption.Text"=w334) -> ()  [unwired: 2 in, 2 out]
          }
          frame "Compressor", "Digital Out" {
            w342 = FALSE ("Visible")
            # "Get direction and finish"
            n189 = property on="Motor" class="Clust (strict)"("Visible"=w342) -> ()  [unwired: 2 in, 2 out]
            n190 = property on="Test Slider" class="Slide (strict)"("Visible"=w342) -> ()  [unwired: 2 in, 2 out]
            n191 = property on="Test Ring" class="Ring (strict)"("Visible"=w342) -> ()  [unwired: 2 in, 2 out]
            n192 = property on="On/Off" class="Bool (strict)"("Visible"=TRUE, "Caption.Text"=w343) -> ()  [unwired: 2 in, 2 out]
            n193 = property on="Rev/Fwd" class="Clust (strict)"("Visible"=FALSE) -> ()  [unwired: 2 in, 2 out]
          }
          frame "Camera" {
            n194 = call <vilib>:"Get Last Path Segment.vi"("String in"=w350) -> ("String out"=w351:string)  [unwired: 10 in]
            n195 = property on="On/Off" class="Bool (strict)"("Visible"=FALSE) -> ()  [unwired: 2 in, 2 out]
            n196 = property on="Motor" class="Clust (strict)"("Visible"=FALSE) -> ()  [unwired: 2 in, 2 out]
            n197 = property on="Rev/Fwd" class="Clust (strict)"("Visible"=FALSE) -> ()  [unwired: 2 in, 2 out]
            n198 = case shown="\"White Balance  **\"" w351 {
              tunnel: w350 -> [w357 w366 w375 w384 w393 _ w399]
              tunnel: w349 -> [w355 w363 w372 w381 w390 _ _]
              frame "Size  **" {
                n199 = Index Array(array=w355) -> (element=w354:cluster{string[]})  [unwired: 1 in]
                n200 = call <vilib>:"NT Read String.vi"("Name"=w357) -> ("String"=w356:string)  [unwired: 9 in, 1 out]
                n201 = Unbundle(w354) -> (w352:string[])
                n202 = Match First String(2:w352, 3:w356) -> (0:w353:i32)  [unwired: 1 out]
                n203 = property on="Test Ring" class="Ring (strict)"("Value"=w353, "Strings []"=w352) -> ()  [unwired: 2 in, 2 out]
                n204 = property on="Test Ring" class="Ring (strict)"("Visible"=TRUE) -> ()  [unwired: 2 in, 2 out]
                n205 = property on="Test Slider" class="Slide (strict)"("Visible"=FALSE) -> ()  [unwired: 2 in, 2 out]
              }
              frame "White Balance  **" {
                n206 = Index Array(array=w363, index=1) -> (element=w364:cluster{string[]})
                n207 = call <vilib>:"NT Read String.vi"("Name"=w366) -> ("String"=w365:string)  [unwired: 9 in, 1 out]
                n208 = Unbundle(w364) -> (w361:string[])
                n209 = Match First String(2:w361, 3:w365) -> (0:w360:i32)  [unwired: 1 out]
                n210 = property on="Test Ring" class="Ring (strict)"("Value"=w360, "Strings []"=w361) -> ()  [unwired: 2 in, 2 out]
                n211 = property on="Test Ring" class="Ring (strict)"("Visible"=TRUE) -> ()  [unwired: 2 in, 2 out]
                n212 = property on="Test Slider" class="Slide (strict)"("Visible"=FALSE) -> ()  [unwired: 2 in, 2 out]
              }
              frame "Exposure  **" {
                n213 = Index Array(array=w372, index=2) -> (element=w373:cluster{string[]})
                n214 = call <vilib>:"NT Read String.vi"("Name"=w375) -> ("String"=w374:string)  [unwired: 9 in, 1 out]
                n215 = Unbundle(w373) -> (w369:string[])
                n216 = Match First String(2:w369, 3:w374) -> (0:w370:i32)  [unwired: 1 out]
                n217 = property on="Test Ring" class="Ring (strict)"("Value"=w370, "Strings []"=w369) -> ()  [unwired: 2 in, 2 out]
                n218 = property on="Test Ring" class="Ring (strict)"("Visible"=TRUE) -> ()  [unwired: 2 in, 2 out]
                n219 = property on="Test Slider" class="Slide (strict)"("Visible"=FALSE) -> ()  [unwired: 2 in, 2 out]
              }
              frame "Exposure Priority  **" {
                n220 = Index Array(array=w381, index=3) -> (element=w382:cluster{string[]})
                n221 = call <vilib>:"NT Read String.vi"("Name"=w384) -> ("String"=w383:string)  [unwired: 9 in, 1 out]
                n222 = Unbundle(w382) -> (w378:string[])
                n223 = Match First String(2:w378, 3:w383) -> (0:w379:i32)  [unwired: 1 out]
                n224 = property on="Test Ring" class="Ring (strict)"("Value"=w379, "Strings []"=w378) -> ()  [unwired: 2 in, 2 out]
                n225 = property on="Test Ring" class="Ring (strict)"("Visible"=TRUE) -> ()  [unwired: 2 in, 2 out]
                n226 = property on="Test Slider" class="Slide (strict)"("Visible"=FALSE) -> ()  [unwired: 2 in, 2 out]
              }
              frame "Color Enable  **" {
                n227 = Index Array(array=w390, index=4) -> (element=w391:cluster{string[]})
                n228 = call <vilib>:"NT Read String.vi"("Name"=w393) -> ("String"=w392:string)  [unwired: 9 in, 1 out]
                n229 = Unbundle(w391) -> (w387:string[])
                n230 = Match First String(2:w387, 3:w392) -> (0:w388:i32)  [unwired: 1 out]
                n231 = property on="Test Ring" class="Ring (strict)"("Value"=w388, "Strings []"=w387) -> ()  [unwired: 2 in, 2 out]
                n232 = property on="Test Ring" class="Ring (strict)"("Visible"=TRUE) -> ()  [unwired: 2 in, 2 out]
                n233 = property on="Test Slider" class="Slide (strict)"("Visible"=FALSE) -> ()  [unwired: 2 in, 2 out]
              }
              frame Default {
                n234 = property on="Test Ring" class="Ring (strict)"("Visible"=FALSE) -> ()  [unwired: 2 in, 2 out]
                n235 = property on="Test Slider" class="Slide (strict)"("Visible"=FALSE) -> ()  [unwired: 2 in, 2 out]
              }
              frame "Brightness  **", "Color Level  **", "Compression  **", "FPS  **", "Sharpness  **" {
                n236 = call <vilib>:"NT Read Number.vi"("Name"=w399) -> ("Numeric"=w398:dbl)  [unwired: 9 in, 1 out]
                n237 = local write "Test Slider"(w398) -> ()
                n238 = property on="Test Slider" class="Slide (strict)"("Visible"=TRUE, "Scale.Maximum"=100.0 ("Scale.Range:Maximum")) -> ()  [unwired: 2 in, 2 out]
                n239 = property on="Test Ring" class="Ring (strict)"("Visible"=FALSE) -> ()  [unwired: 2 in, 2 out]
              }
            }
          }
        }
        n240 = property on="Progress" class="Clust (strict)"("Visible"=FALSE) -> ()  [unwired: 2 in, 2 out]
      }
      event "Test Name": Mouse Enter {
        # "Populate the ring with the list of tests"
        n241 = event-data() -> ()  [unwired: 1 in, 1 out]
        n242 = call <vilib>:"NT Read String Array.vi"("Name"="TestMode/TestList") -> ("String Array"=w407:string[])  [unwired: 9 in, 1 out]
        n243 = Build Array (concatenate)("Select the test to run...", w407) -> (w406:string[])
        n244 = property on="Test Name" class="Ring (strict)"("Strings []"=w406) -> ()  [unwired: 2 in, 2 out]
      }
      event "Test Name": Value Change {
        w409 = FALSE ("Visible")
        # "Tell the robot the test name to run"
        n245 = event-data() -> ("NewVal"=w413:u16)  [unwired: 1 in]
        n246 = property on="Test Name" class="Ring (strict)"() -> ("Strings []"=w414:string[])  [unwired: 2 in, 2 out]
        n247 = local write "Progress"(T9 {"Test Progress"=0, "Test Progress Text"=""} ("Progress")) -> ()
        n248 = Index Array(array=w414, index=w413) -> (element=w412:string)
        n249 = call <vilib>:"NT Write String.vi"("String"=w412, "Name"="TestMode/TestName") -> ()  [unwired: 9 in, 1 out]
        n250 = property on="Progress" class="Clust (strict)"("Visible"=TRUE) -> ()  [unwired: 2 in, 2 out]
        n251 = property on="Motor" class="Clust (strict)"("Visible"=w409) -> ()  [unwired: 2 in, 2 out]
        n252 = property on="Test Slider" class="Slide (strict)"("Visible"=w409) -> ()  [unwired: 2 in, 2 out]
        n253 = property on="On/Off" class="Bool (strict)"("Visible"=w409) -> ()  [unwired: 2 in, 2 out]
        n254 = property on="Rev/Fwd" class="Clust (strict)"("Visible"=w409) -> ()  [unwired: 2 in, 2 out]
        n255 = property on="Test Ring" class="Ring (strict)"("Visible"=w409) -> ()  [unwired: 2 in, 2 out]
      }
      event "Select Auto": Mouse Enter {
        # "Populate the combo box with the list of autonomous options"
        n256 = event-data() -> ()  [unwired: 1 in, 1 out]
        n257 = call <vilib>:"NT Read String Array.vi"("Name"="Auto List") -> ("String Array"=w416:string[])  [unwired: 9 in, 1 out]
        n258 = property on="Select Auto" class="CmbBox"("Strings[]"=w416) -> ()  [unwired: 2 in, 2 out]
      }
      event "Select Auto": Value Change {
        # "User modified the Auto Selection. Write to NT variable so robot knows."
        n259 = event-data() -> ("NewVal"=w419:string)  [unwired: 1 in]
        n260 = call <vilib>:"NT Write String.vi"("String"=w419, "Name"="Auto Selector") -> ()  [unwired: 9 in, 1 out]
      }
      event "Command Selection": Value Change {
        # "Get the params and show in table"
        n261 = event-data() -> ("NewVal"=w425:i32)  [unwired: 1 in]
        n262 = property on="Command Selection" class="MCListbox (strict)"() -> ("ItemNames"=w423:string[][])  [unwired: 2 in, 2 out]
        n263 = call <vilib>:"WPI_DashboardUpdate Command Params.vi"("NewVal"=w425, "Commands"=w423, "Param Tbl"=w424) -> ()  [unwired: 8 in, 1 out]
      }
      event "Execute Command": Value Change {
        # "Started one, Unique ID holds\nresponse"
        n264 = event-data() -> ()  [unwired: 1 in, 1 out]
        n265 = property on="Command Selection" class="MCListbox (strict)"() -> ("ItemNames"=w436:string[][])  [unwired: 2 in, 2 out]
        n266 = Index Array(array=w436, index (row)="Command Selection", index (col)=0) -> (element=w434:string)
        n267 = call <vilib>:"Invoke Commands.vi"("Command Params"="Command Params", "Function Name"=w434) -> ("Params"=w430:u8, "Started"=w429:bool)  [unwired: 7 in, 1 out]
        n268 = Array Subset(array="Command Params", length (row)=w430) -> (w431:string[][])  [unwired: 3 in]
        n269 = Select(t="Executing" ("Cmd Status"), s=w429, f="" ("Cmd Status")) -> (s? t:f=→"Cmd Status":string)
      }
      event "Command Selection": Double Click {
        n270 = event-data() -> ("Row"=w444:i32)  [unwired: 1 in]
        n271 = property on="Command Selection" class="MCListbox (strict)"() -> ("ItemNames"=w447:string[][])  [unwired: 2 in, 2 out]
        n272 = local read "Command Params"() -> (w443:string[][])
        n273 = Index Array(array=w447, index (row)=w444, index (col)=0) -> (element=w445:string)
        n274 = call <vilib>:"Invoke Commands.vi"("Command Params"=w443, "Function Name"=w445) -> ("Params"=w442:u8, "Started"=w437:bool)  [unwired: 7 in, 1 out]
        n275 = Array Subset(array=w443, length (row)=w442) -> (w441:string[][])  [unwired: 3 in]
        n276 = Select(t="Executing" ("Cmd Status"), s=w437, f="" ("Cmd Status")) -> (s? t:f=w438:string)
        n277 = local write "Cmd Status"(w438) -> ()
      }
      event "CheckList": Double Click {
        # "Shift clears all"
        # "Update symbols on the listbox"
        n278 = event-data() -> ("PlatMods.Shift"=w449:bool, "Row"=w451:i32)  [unwired: 1 in]
        n279 = case shown="True" w449 {
          tunnel: w451 -> [w455 _]
          tunnel: 1 -> [w454 _]
          frame False {
            n280 = property on="CheckList" class="LstBox (strict)"() -> ("Item Symbols"=w453:i32[])  [unwired: 2 in, 2 out]
            n281 = Replace Array Subset(array=w453, new element=w454, index=w455) -> (w452:i32[])
            n282 = property on="CheckList" class="LstBox (strict)"("Item Symbols"=w452) -> ()  [unwired: 2 in, 2 out]
          }
          frame True {
            w456 = 0 ("Top Row")
            n283 = property on="CheckList" class="LstBox (strict)"() -> ("Number of Rows"=w458:u32)  [unwired: 2 in, 2 out]
            n284 = Initialize Array(0, w458) -> (w457:i32[])
            n285 = property on="CheckList" class="LstBox (strict)"("Top Row"=w456, "Value"=w456, "Item Symbols"=w457) -> ()  [unwired: 2 in, 2 out]
          }
        }
      }
      event "CheckList": Key Down {
        # "Update symbols on the listbox\nLeft and right keys check and uncheck"
        n286 = event-data() -> ("VKey"=w462:T25)  [unwired: 1 in]
        n287 = case shown="\"Left\", \"Right\"" w462 {
          selector: w462 -> [w467 _]
          tunnel: eventvkey."Left" ("VKey") -> [w465 _]
          frame "Left", "Right" {
            n288 = Equal?(x=w465, y=w467) -> (x = y?=w466:bool)
            n289 = Select(t=0, s=w466, f=1) -> (s? t:f=w468:i32)
            n290 = property on="CheckList" class="LstBox (strict)"() -> ("Item Symbols"=w471:i32[])  [unwired: 2 in, 2 out]
            n291 = Replace Array Subset(array=w471, new element=w468, index="CheckList") -> (w470:i32[])
            n292 = property on="CheckList" class="LstBox (strict)"("Item Symbols"=w470) -> ()  [unwired: 2 in, 2 out]
          }
          frame Default {
          }
        }
      }
      event "Motor.Enable": Value Change {
        # "When the test mode otor enable helper is set, update that\ntree row item's value"
        n293 = event-data() -> ("NewVal"=w477:bool)  [unwired: 1 in]
        n294 = Unbundle("Motor") -> ("Value"=w476:dbl)  [unwired: 1 out]
        n295 = Select(t=w476, s=w477, f=0.0) -> (s? t:f=w474:dbl)
        n296 = call <vilib>:"NT Write Number.vi"("Numeric"=w474, "Name"=w473) -> ()  [unwired: 9 in, 1 out]
      }
      event "Test Slider": Value Change {
        # "When the test mode slider helper is set, update that\ntree row item's value"
        n297 = event-data() -> ("NewVal"=w480:dbl)  [unwired: 1 in]
        n298 = call <vilib>:"NT Write Number.vi"("Numeric"=w480, "Name"=w481) -> ()  [unwired: 9 in, 1 out]
      }
      event "On/Off": Value Change {
        # "When the test mode on/off helper value is set, update that\ntree row item's value"
        n299 = event-data() -> ("NewVal"=w485:bool)  [unwired: 1 in]
        n300 = Boolean To (0,1)(Boolean=w485) -> (0, 1=w484:i16)
        n301 = call <vilib>:"NT Write Number.vi"("Numeric"=w484, "Name"=w483) -> ()  [unwired: 9 in, 1 out]
      }
      event "Rev/Fwd": Value Change {
        # "When the test mode helper value for relays is set, update that\ntree row item's value"
        n302 = event-data() -> ("NewVal.Forward"=w493:bool, "NewVal.Reverse"=w492:bool)  [unwired: 1 in]
        n303 = Boolean To (0,1)(Boolean=w493) -> (0, 1=w489:i16)
        n304 = Boolean To (0,1)(Boolean=w492) -> (0, 1=w491:i16)
        n305 = Negate(x=w491) -> (-x=w490:i16)
        n306 = Add(x=w489, y=w490) -> (x+y=w488:i16)
        n307 = call <vilib>:"NT Write Number.vi"("Numeric"=w488, "Name"=w487) -> ()  [unwired: 9 in, 1 out]
      }
      event "Test Ring": Value Change {
        # "When a test mode helper value is selected from the ring,\nset the tree item's variable to the string value"
        n308 = event-data() -> ("NewVal"=w497:u16)  [unwired: 1 in]
        n309 = property on="Test Ring" class="Ring (strict)"() -> ("Strings []"=w498:string[])  [unwired: 2 in, 2 out]
        n310 = Index Array(array=w498, index=w497) -> (element=w496:string)
        n311 = call <vilib>:"NT Write String.vi"("String"=w496, "Name"=w495) -> ()  [unwired: 9 in, 1 out]
      }
      event "Rec Mode": Value Change {
        # "Update globals for recording mode and path to read log from.\nClear when logging and let NetworkTables set path for vision to\nuse."
        n312 = event-data() -> ("NewVal"=w509:enum32{"Stop", "Record", "Playback"})  [unwired: 1 in]
        n313 = global write "WPI_DashboardLogging Global.vi" "Logging Filename"(path "") -> ()
        n314 = global write "WPI_DashboardLogging Global.vi" "Recording"(w509) -> ()
        n315 = case shown="\"Playback\"" w509 {
          tunnel: w508 -> [_ w511 w520]
          tunnel: [_ _ w519] -> w506
          tunnel: [_ _ w518] -> _
          tunnel: w504 -> [_ _ w516]
          tunnel: cluster{i32, i32} {-250, 170} -> [_ _ w515]
          tunnel: [_ _ T26 {"Image Size"=TRUE, "Image Type"=TRUE, "Pixel Value"=TRUE, "ROI Information"=TRUE, "Zoom Factor"=FALSE} ("Image Information Shown:All Elements")] -> w499
          tunnel: [_ _ TRUE ("Zoom Factor")] -> w500
          tunnel: w502 -> [_ _ w512]
          frame Default {
          }
          frame "Stop", "Record" {
            # "Place Window too"
            n316 = invoke class="VI" method="FP.Close"(reference=w511) -> (reference out=w510:refnum<vi>)  [unwired: 2 in, 2 out]
            n317 = invoke class="VI" method="Abort VI"(reference=w510) -> ()  [unwired: 2 in, 3 out]
          }
          frame "Playback" {
            n318 = call "Open Playback Panel.vi"("Offset"=w515, "DB VI Ref"=w516, "Playback in"=w520) -> ("Playback out"=w517:refnum<vi>)  [unwired: 8 in]
            n319 = register-events(w517, w512) -> (reference out=w519:refnum<event-registration>, error out=w518:errorcluster)  [unwired: 2 in]
          }
        }
        n320 = property on="Camera Image Right" class="ImageControl"("Image Information Shown"=w499, "Image Information Visible"=w500) -> ()  [unwired: 2 in, 2 out]
        n321 = property on="Camera Image" class="ImageControl"("Image Information Shown"=w499, "Image Information Visible"=w500) -> ()  [unwired: 2 in, 2 out]
        n322 = call <vilib>:"WPI_DashboardNT Log FieldName Cache.vi"("Operation"=enum16{"Lookup/Add", "Index", "Clear"}."Clear") -> ()  [unwired: 8 in, 3 out]
      }
      event Panel Close {
        w522 = enum32{"Stop", "Record", "Playback"}."Stop" ("Rec Mode")
        # "Playback window has been closed, abort"
        n323 = event-data() -> ()  [unwired: 1 in, 4 out]
        n324 = local write "Rec Mode"(w522) -> ()
        n325 = global write "WPI_DashboardLogging Global.vi" "Recording"(w522) -> ()
      }
      event Panel Close {
        # "Abort playback window and ourself"
        n326 = event-data() -> ()  [unwired: 1 in, 4 out]
        n327 = invoke class="VI" method="FP.Close"(reference=w526) -> (reference out=w525:refnum<vi>)  [unwired: 2 in, 2 out]
        n328 = invoke class="VI" method="Abort VI"(reference=w525) -> (error out=w524:errorcluster)  [unwired: 2 in, 2 out]
        n329 = invoke class="VI" method="Abort VI"(error in=w524) -> ()  [unwired: 2 in, 3 out]
      }
      event User Event {
        n330 = event-data() -> ("IDs"=w533:cluster{"RPC field ID":u16, "Unique ID":u16}, "String"=w532:string)  [unwired: 1 in]
        n331 = Bundle("IDs"=w533, "String"=w532) -> (w531:T12)  [unwired: 1 in]
        n332 = call <vilib>:"Retrieve RPC Response.vi"("RPC Response"=w531) -> ("Output"=w529:string[][])  [unwired: 10 in]
        n333 = Build Array (concatenate)(w527, w529) -> (w528:string[][])
        n334 = local write "Command Params"(w528) -> ()
        n335 = local write "Cmd Status"("" ("Cmd Status")) -> ()
      }
      event "Tree": Double Click {
        n336 = event-data() -> ("PlatMods"=w539:T29, "Tag"=w536:string)  [unwired: 1 in]
        n337 = Unbundle(w539) -> ("Shift"=w538:bool)  [unwired: 4 out]
        n338 = String Subset(string=w536, length (rest)=1 ("length (rest)")) -> (substring=w535:string)  [unwired: 1 in]
        n339 = Not(x=w538) -> (.not. x?=w537:bool)
        n340 = case shown="\"/\"" w535 {
          tunnel: w536 -> [_ w542]
          tunnel: w537 -> [_ w541]
          frame Default {
          }
          frame "/" {
            n341 = call <vilib>:"NT Update Persistence.vi"("Persistence"=w541, "Name"=w542) -> ()  [unwired: 9 in, 1 out]
          }
        }
      }
    }
  }
  n342 = while {
    tunnel: w65 -> [w544]
    i -> [w547]
    stop <- FALSE stop-if-true
    n343 = Wait (ms)(milliseconds to wait=u32 100) -> ()  [unwired: 1 out]
    n344 = case shown="\"Playback\"" "Rec Mode" {
      tunnel: w547 -> [_ _ w562]
      tunnel: [u32 2829099 ("Base Color") u32 11141120 ("Target Color") w551] -> w543
      frame "Stop", Default {
        # "Reset the color, extra updates don't cost much"
      }
      frame "Record" {
      }
      frame "Playback" {
        # "Playback"
        n345 = Quotient & Remainder(x=w562, y=u32 50 ("milliseconds to wait")) -> (x-y*floor(x/y)=w558:u32)  [unwired: 1 out]
        n346 = Divide(x=w558, y=u32 50 ("milliseconds to wait")) -> (x/y=w555:dbl)
        n347 = Multiply(x=6.283185307179586, y=w555) -> (x*y=w560:dbl)
        n348 = Sine(x=w560) -> (sin(x)=w559:dbl)
        n349 = Absolute Value(x=w559) -> (abs(x)=w552:dbl)
        n350 = call "Interpolate RGB Color.vi"("Proportion"=w552, "Target Color"=u32 30976, "Base Color"=u32 2829099) -> ("Result Color"=w551:u32)  [unwired: 8 in]
      }
    }
    n351 = property class="Pane"(reference=w544, "PaneColor"=w543) -> ()  [unwired: 1 in, 2 out]
  }
  n352 = while {
    stop <- FALSE stop-if-true
    n353 = Wait (ms)(milliseconds to wait=u32 300) -> ()  [unwired: 1 out]
    n354 = call-poly <vilib>:"NT Write Value.vi"("String"="Battery Number", "Name"="BatteryNumber") -> ()  [unwired: 9 in, 1 out]
    n355 = Get Date/Time In Seconds() -> (seconds since 1Jan1904=w564:timestamp)
    n356 = Format Date/Time String(time format string (%c)="%Y.%m.%d.%H.%M", seconds (now)=w564) -> (date/time string=w563:string)  [unwired: 1 in]
    n357 = call-poly <vilib>:"NT Write Value.vi"("String"=w563, "Name"="DateandTime") -> ()  [unwired: 9 in, 1 out]
  }
  n358 = local write "Dashboard Tab"(T2."Drive" ("Dashboard Tab")) -> ()
  n359 = property on="On/Off" class="Bool (strict)"("Visible"=w36) -> ()  [unwired: 2 in, 2 out]
  n360 = property on="Motor" class="Clust (strict)"("Visible"=w36) -> ()  [unwired: 2 in, 2 out]
  n361 = property on="Progress" class="Clust (strict)"("Visible"=w36) -> ()  [unwired: 2 in, 2 out]
  n362 = property on="Test Ring" class="Ring (strict)"("Visible"=w36) -> ()  [unwired: 2 in, 2 out]
  n363 = property on="Rev/Fwd" class="Clust (strict)"("Visible"=w36) -> ()  [unwired: 2 in, 2 out]
  n364 = while {
    tunnel: u16 1741 ("timeout ms (25000)") -> [w572]
    stop <- FALSE stop-if-true
    n365 = TCP Create Listener(10:w572) -> (0:w571:errorcluster, 3:w573:refnum<k5>)  [unwired: 4 in, 1 out]
    n366 = case shown="No Error" w571 {
      selector: w571 -> [w575 _]
      tunnel: w573 -> [w576 _]
      frame No Error {
        n367 = while {
          tunnel: w576 -> [w579]
          tunnel: w575 -> [w578]
          stop <- FALSE stop-if-true
          n368 = TCP Wait On Listener(8:w578, 11:w579) -> (0:w580:errorcluster, 4:w581:refnum<k5>)  [unwired: 2 in, 3 out]
          n369 = local write "TCP"(w581) -> ()
          n370 = case shown="No Error" w580 {
            frame No Error {
            }
            frame Error {
              n371 = Wait (ms)(milliseconds to wait=u32 1000) -> ()  [unwired: 1 out]
            }
          }
        }
      }
      frame Error {
        n372 = Wait (ms)(milliseconds to wait=u32 1000) -> ()  [unwired: 1 out]
      }
    }
  }
  n373 = local write "Command Selection"(u16 0 ("milliseconds to wait")) -> ()
  n374 = local write "Command Params"(string[][] [] ("Command Params")) -> ()
  n375 = global write "WPI_DashboardLogging Global.vi" "Recording"(w59) -> ()
  n376 = local write "Rec Mode"(w59) -> ()
  n377 = call <vilib>:"NT Write String.vi"("String"="Select Auto", "Name"="Auto Selector") -> ()  [unwired: 9 in, 1 out]
